vi "VIG - Get Update Coordinates.vi"(7 "Pane Method":T1, 8 "error in (no error)":errorcluster, 10 "MasterRect":T4, 11 "Pane in":refnum<vi>) -> (0 "error out":errorcluster, 2 "Offset From Start":T2, 3 "Coordinates":T3)   [LabVIEW 2017, in "Front Panel Publisher.lvlib" / "Object.lvclass"]
uses:
  Object.lvclass
  Coordinates.ctl
  <vilib>/Utility/miscctls.llb/LVPointTypeDef.ctl
  <vilib>/Utility/miscctls.llb/LVRectTypeDef.ctl
  Enum - Pane Coordinate Method.ctl
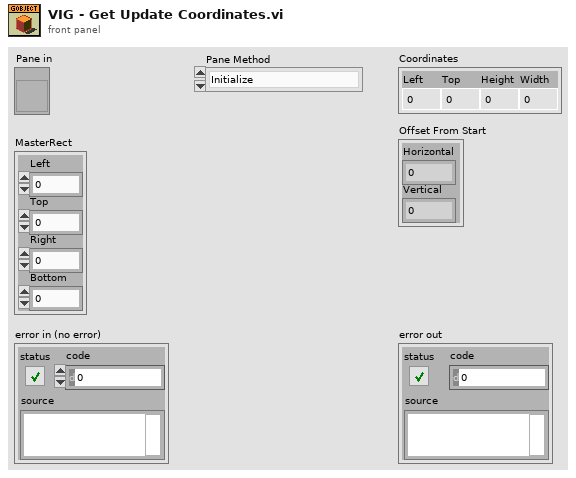
[diagram p1: front panel]
types:
  T1 = typedef "Front Panel Publisher.lvlib/Object.lvclass/Enum - Pane Coordinate Method.ctl" = enum16{"Initialize", "Get Last Pane Offset", "Update Pane Position"}
  T2 = typedef "LVPointTypeDef.ctl" = cluster{"Horizontal":i16, "Vertical":i16}
  T3 = typedef "Front Panel Publisher.lvlib/Object.lvclass/Coordinates.ctl" = cluster{"Left":i32, "Top":i32, "Height":u32, "Width":u32}
  T4 = typedef "LVRectTypeDef.ctl" = cluster{"Left":i16, "Top":i16, "Right":i16, "Bottom":i16}
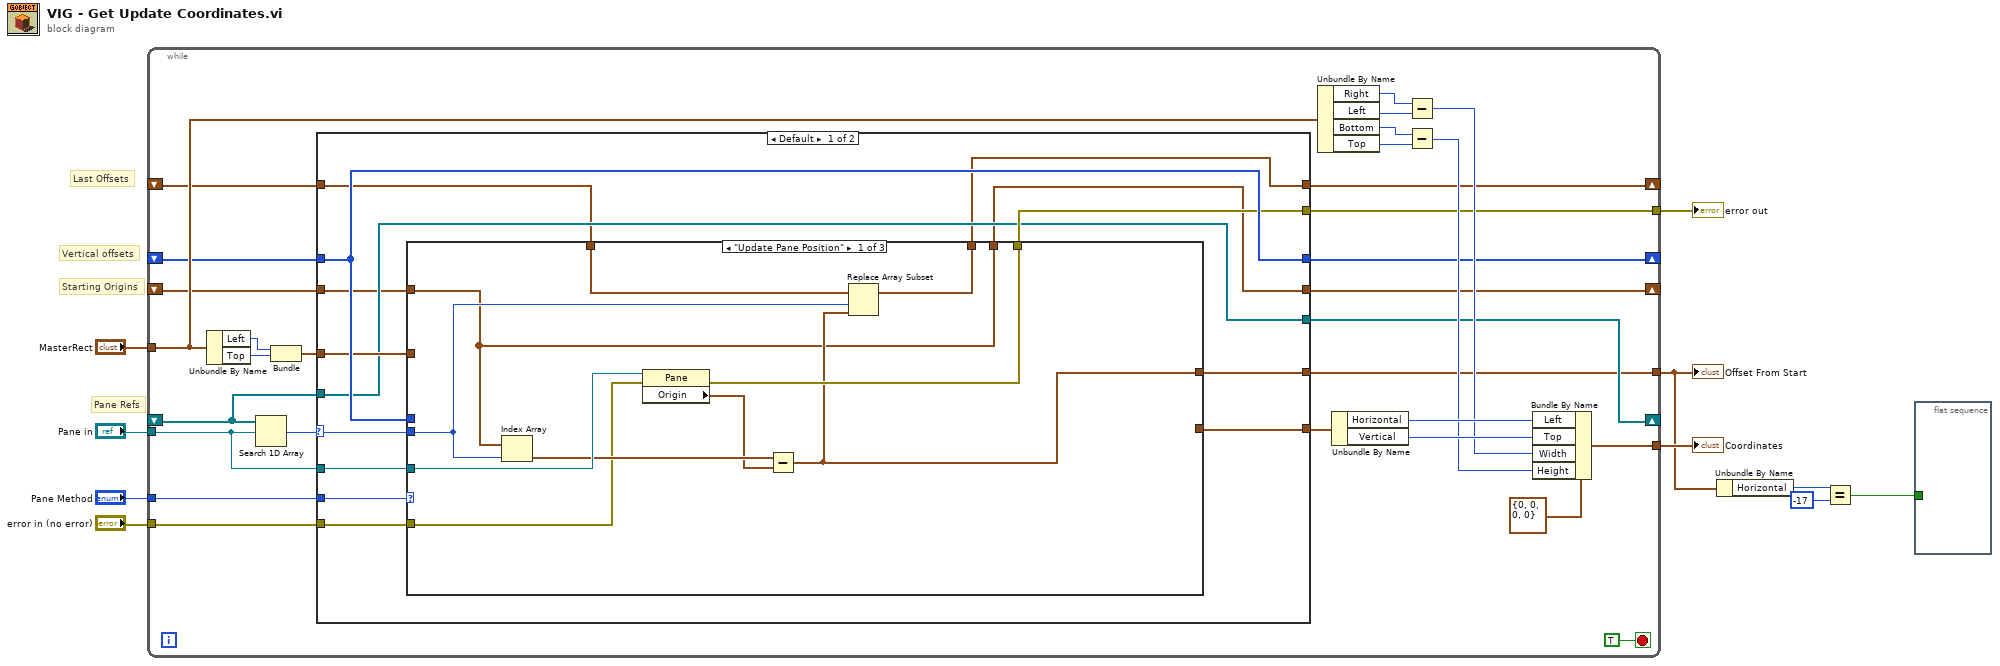
[diagram p0: block diagram]
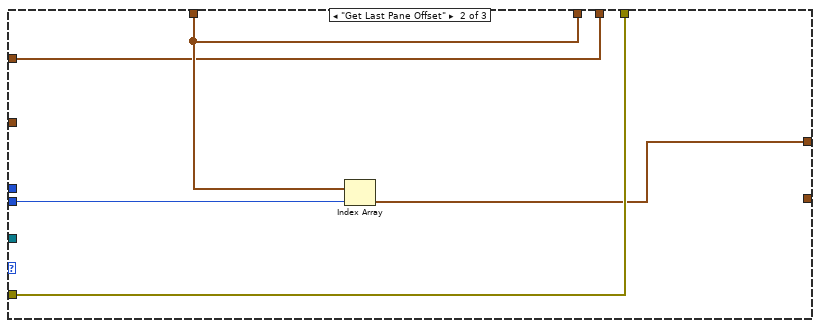
[diagram p2: hidden frame]
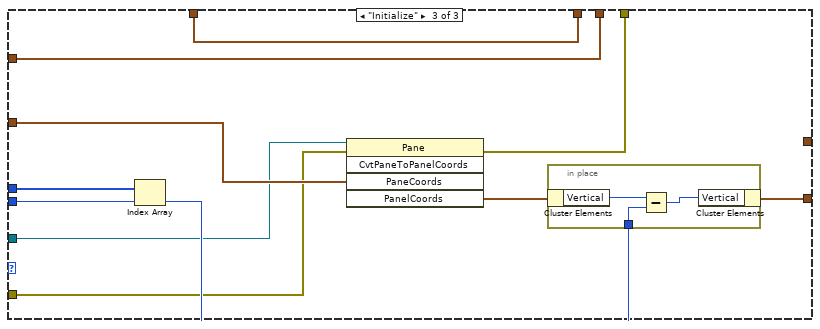
[diagram p3: hidden frame]
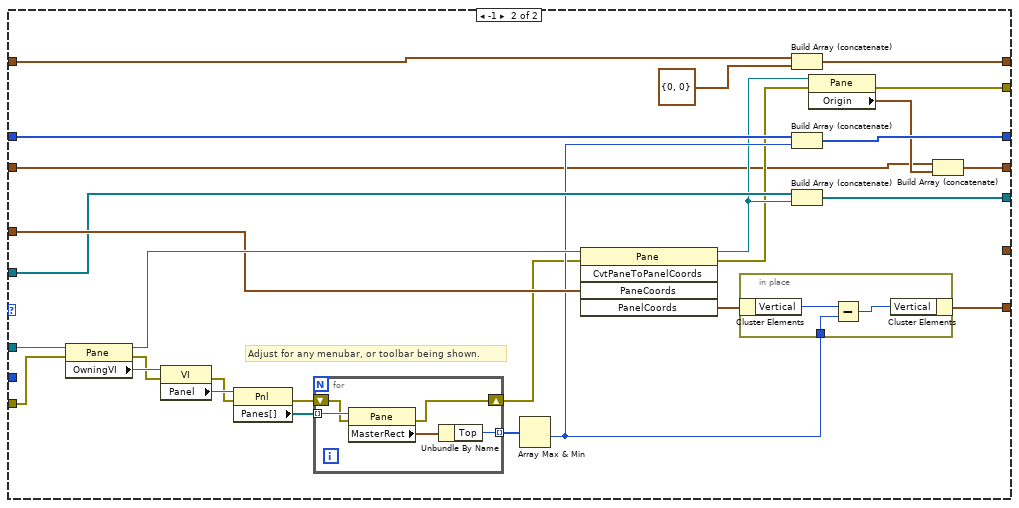
[diagram p4: hidden frame]
diagram:
  # "Last Offsets"
  # "Pane Refs"
  # "Starting Origins"
  # "Vertical offsets"
  n1 = while {
    tunnel: [w40] -> w5
    tunnel: "Pane in" -> [w35]
    shift-right: [w21] -> _
    shift-left: _ -> [w22]
    tunnel: "MasterRect" -> [w30]
    shift-right: [w20] -> _
    shift-left: _ -> [w19]
    shift-right: [w18] -> _
    shift-left: _ -> [w17]
    tunnel: "error in (no error)" -> [w16]
    tunnel: [w15] -> w7
    tunnel: [w14] -> w4
    tunnel: "Pane Method" -> [w13]
    shift-right: [w12] -> _
    shift-left: _ -> [w11]
    stop <- TRUE stop-if-true
    n2 = Unbundle By Name(w30) -> ("Left"=w33:i16, "Top"=w34:i16)
    n3 = Search 1D Array(1D array=w22, element=w35) -> (index of element=w36:i32)  [unwired: 1 in]
    n4 = Bundle("Left"=w33, "Top"=w34) -> (w32:cluster{"Left":i16, "Top":i16})  [unwired: 1 in]
    n5 = case shown="Default" w36 {
      selector: w36 -> [w53 _]
      tunnel: w35 -> [w51 w111]
      tunnel: w32 -> [w52 w101]
      tunnel: [w50 w100] -> w31
      tunnel: w22 -> [w47 w99]
      tunnel: [w47 w98] -> w21
      tunnel: [w54 w96] -> w20
      tunnel: w19 -> [w54 w95]
      tunnel: [w42 w90] -> w18
      tunnel: w17 -> [w41 w89]
      tunnel: [w49 w88] -> w15
      tunnel: w16 -> [w48 w87]
      tunnel: [w46 _] -> w14
      tunnel: w13 -> [w45 _]
      tunnel: [w44 w85] -> w12
      tunnel: w11 -> [w43 w84]
      frame Default {
        n6 = case shown="\"Update Pane Position\"" w45 {
          tunnel: w54 -> [_ _ w80]
          tunnel: w53 -> [w56 w69 w79]
          tunnel: w52 -> [_ _ w76]
          tunnel: w51 -> [w64 _ w75]
          tunnel: [_ _ w74] -> w50
          tunnel: [w62 w67 w73] -> w49
          tunnel: w48 -> [w61 w67 w72]
          tunnel: w41 -> [w55 w65 w70]
          tunnel: [w58 w66 _] -> w46
          tunnel: w43 -> [w60 w68 w71]
          tunnel: [w59 w68 w71] -> w44
          tunnel: [w55 w65 w70] -> w42
          frame "Update Pane Position" {
            n7 = Index Array(array=w55, index=w56) -> (element=w63:T2)
            n8 = property class="Pane"(reference=w64, error in=w61) -> (error out=w62:errorcluster, "Origin"=w57:T2)  [unwired: 1 out]
            n9 = Subtract(x=w63, y=w57) -> (x-y=w58:T2)
            n10 = Replace Array Subset(array=w60, new element=w58, index=w56) -> (w59:T2[])
          }
          frame "Get Last Pane Offset" {
            n11 = Index Array(array=w68, index=w69) -> (element=w66:T2)
          }
          frame "Initialize" {
            n12 = Index Array(array=w80, index=w79) -> (element=w77:i16)
            n13 = invoke class="Pane" method="CvtPaneToPanelCoords"(reference=w75, error in=w72, "PaneCoords"=w76) -> (error out=w73:errorcluster, "PanelCoords"=w78:T2)  [unwired: 2 in, 3 out]
            n14 = in-place {
              in-place-border: w77 -> [w82]
              n15 = in-place-cluster #1(w78) -> ("Vertical"=w83:i16)
              n16 = Subtract(x=w83, y=w82) -> (x-y=w81:i16)
              n17 = in-place-cluster #1("Vertical"=w81) -> (w74:T2)
            }
          }
        }
      }
      frame -1 {
        # "Adjust for any menubar, or toolbar being shown."
        n18 = property class="Pane"(reference=w111, error in=w87) -> (reference out=w102:refnum<vi>, error out=w108:errorcluster, "OwningVI"=w109:refnum<vi>)
        n19 = property class="VI"(reference=w109, error in=w108) -> (error out=w107:errorcluster, "Panel"=w110:refnum<vi>)  [unwired: 1 out]
        n20 = property class="Pnl"(reference=w110, error in=w107) -> (error out=w104:errorcluster, "Panes[]"=w105:refnum<vi>[])  [unwired: 1 out]
        n21 = for {
          tunnel: w105 -> [w119] mode=indexing
          tunnel: [w117] -> w106 mode=indexing
          shift-right: [w115] -> w94
          shift-left: w104 -> [w116]
          n22 = property class="Pane"(reference=w119, error in=w116) -> (error out=w115:errorcluster, "MasterRect"=w118:T4)  [unwired: 1 out]
          n23 = Unbundle By Name(w118) -> ("Top"=w117:i16)
        }
        n24 = Array Max & Min(array=w106) -> (min value=w97:i16)  [unwired: 3 out]
        n25 = invoke class="Pane" method="CvtPaneToPanelCoords"(reference=w102, error in=w94, "PaneCoords"=w101) -> (reference out=w93:refnum<vi>, error out=w92:errorcluster, "PanelCoords"=w103:T2)  [unwired: 2 in, 2 out]
        n26 = in-place {
          in-place-border: w97 -> [w113]
          n27 = in-place-cluster #2(w103) -> ("Vertical"=w114:i16)
          n28 = Subtract(x=w114, y=w113) -> (x-y=w112:i16)
          n29 = in-place-cluster #2("Vertical"=w112) -> (w100:T2)
        }
        n30 = Build Array (concatenate)(w84, T2 {"Horizontal"=0, "Vertical"=0} ("x-y")) -> (w85:T2[])
        n31 = Build Array (concatenate)(w95, w97) -> (w96:i16[])
        n32 = Build Array (concatenate)(w99, w93) -> (w98:refnum<vi>[])
        n33 = property class="Pane"(reference=w93, error in=w92) -> (error out=w88:errorcluster, "Origin"=w91:T2)  [unwired: 1 out]
        n34 = Build Array (concatenate)(w89, w91) -> (w90:T2[])
      }
    }
    n35 = Unbundle By Name(w30) -> ("Right"=w29:i16, "Left"=w28:i16, "Bottom"=w26:i16, "Top"=w25:i16)
    n36 = Unbundle By Name(w31) -> ("Horizontal"=w39:i16, "Vertical"=w38:i16)
    n37 = Subtract(x=w29, y=w28) -> (x-y=w27:i16)
    n38 = Subtract(x=w26, y=w25) -> (x-y=w24:i16)
    n39 = Bundle By Name(cluster=T3 {"Left"=0, "Top"=0, "Height"=0, "Width"=0} ("Coordinates"), "Left"=w39, "Top"=w38, "Width"=w27, "Height"=w24) -> (w40:T3)
  }
  "error out" <- w7
  "Coordinates" <- w5
  "Offset From Start" <- w4
  n40 = Unbundle By Name(w4) -> ("Horizontal"=w3:i16)
  n41 = Equal?(x=w3, y=i16 -17) -> (x = y?=w1:bool)
  n42 = flat-sequence {
    tunnel: w1 -> [_]
    frame #0 {
    }
  }
